vi "DT2.vi"(0 "input u(k)":dbl, 2 "Mode":enum16{"s-domain", "Frequency"}(ring), 5 "s-domain":cluster{"G":dbl, "T1":dbl, "T2":dbl}, 9 "frequency":cluster{"Td":dbl, "D":dbl, "f0":dbl}, 13 "initialize":bool) -> (8 "output y(k)":dbl)   [LabVIEW 2022 SP3]
uses:
  <vilib>/addons/Control Design/_Model Construction/Model Typedefs.llb/CD Transfer Function Model (SISO).ctl
  <vilib>/addons/Control Design/_Model Construction/NI_LinSys_Model Typedefs.lvlib
  <vilib>/addons/Control Design/_Model Construction/Model Typedefs.llb/CD General Elements.ctl
  <vilib>/addons/Control Design/_Model Construction/Model Typedefs.llb/CD Transfer Function Model (MIMO).ctl
  <vilib>/Simulation/DiscreteLinear/Implementation/NILVSim Discrete Transfer Function Direct.llb/SIM Discrete Transfer Function Diagram (SISO CD).vi
  <vilib>/Simulation/Implementation/XNodeFramework/SimXNode/SimX.xnode
  <vilib>/addons/Control Design/_Frequency Response Analysis/NI_CD_Frequency Response.lvlib
  <vilib>/addons/Control Design/_Frequency Response Analysis/Frequency Response.llb/Frequency Response subVI/cd_Bode (Transfer Function).vi
  <vilib>/addons/System Identification/Model Typedefs.llb/si_Bode Magnitude Plot.ctl
  <vilib>/addons/System Identification/NI_SysID.lvlib
  <vilib>/addons/System Identification/Model Typedefs.llb/si_Bode Phase Plot.ctl
panel:
  out "Bode Phase Plot":T1
  out "Bode Magnitude Plot":T2
  out "Step Response Graph":cluster{"time":dbl[], dbl[]}[](graph)
  out "S Transf":picture
  out "error out":errorcluster
  in  "error in (no error)":errorcluster
  out "element":T3 {"delay" format="%.4f"; "Denominator" format="%#_3g"; "Numerator" format="%#_3g"}
  out "Z Transf":picture
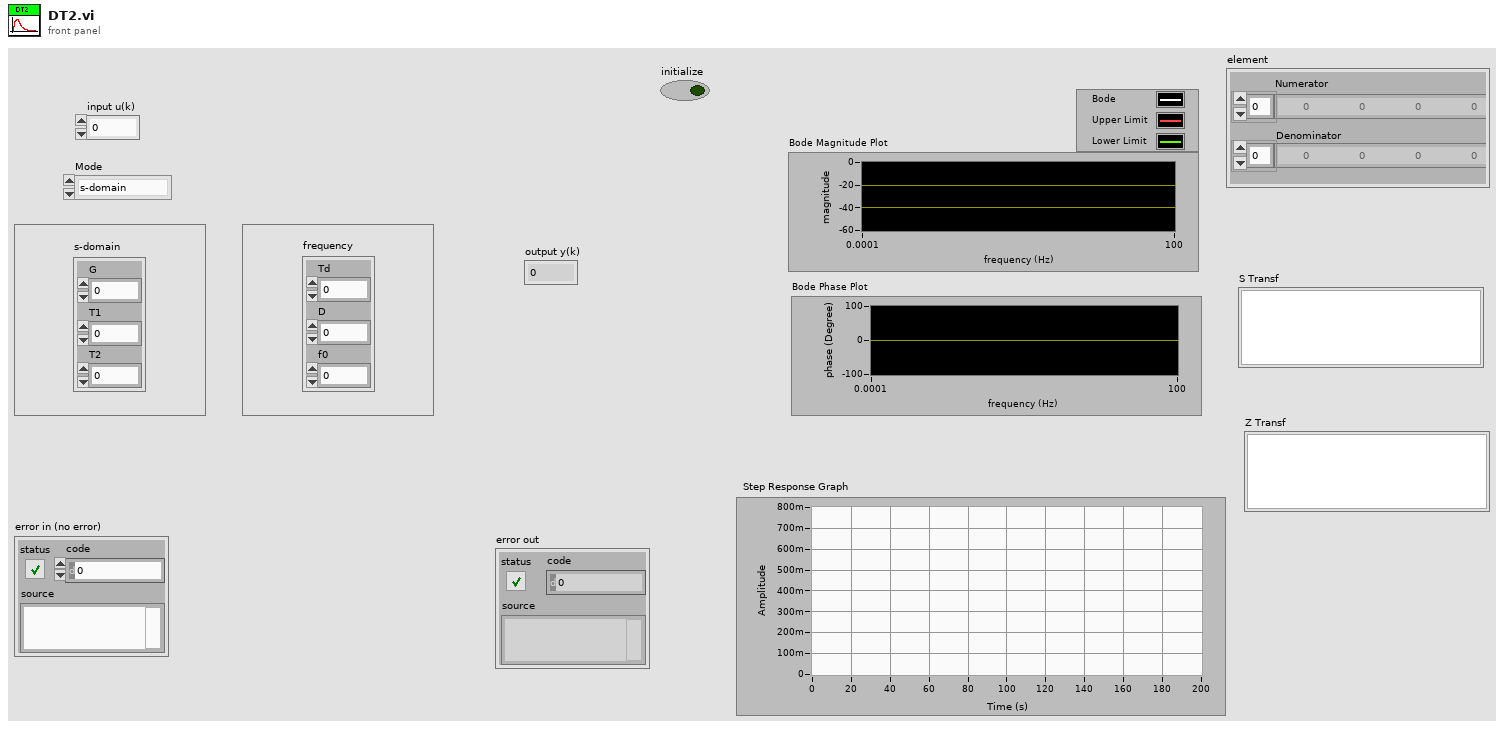
[diagram p1: front panel]
types:
  T1 = typedef "NI_SysID.lvlib/si_Bode Phase Plot.ctl" = cluster{"frequency":dbl[], "amplitude":dbl[]}[]
  T2 = typedef "NI_SysID.lvlib/si_Bode Magnitude Plot.ctl" = cluster{"frequency":dbl[], "amplitude":dbl[]}[]
  T3 = typedef "NI_LinSys_Model Typedefs.lvlib/CD Transfer Function Model (SISO).ctl" = cluster{"Numerator":dbl[], "Denominator":dbl[], "delay":dbl}
  T4 = typedef "NI_LinSys_Model Typedefs.lvlib/CD Transfer Function Model (MIMO).ctl" = cluster{"properties":T5, "transfer function(s)":T3[][]}
  T5 = typedef "NI_LinSys_Model Typedefs.lvlib/CD General Elements.ctl" = cluster{"Model name":string, "Input names":string[], "Output names":string[], "Input Delays":dbl[], "Output Delays":dbl[], "Sampling Time":dbl, "Notes":string}
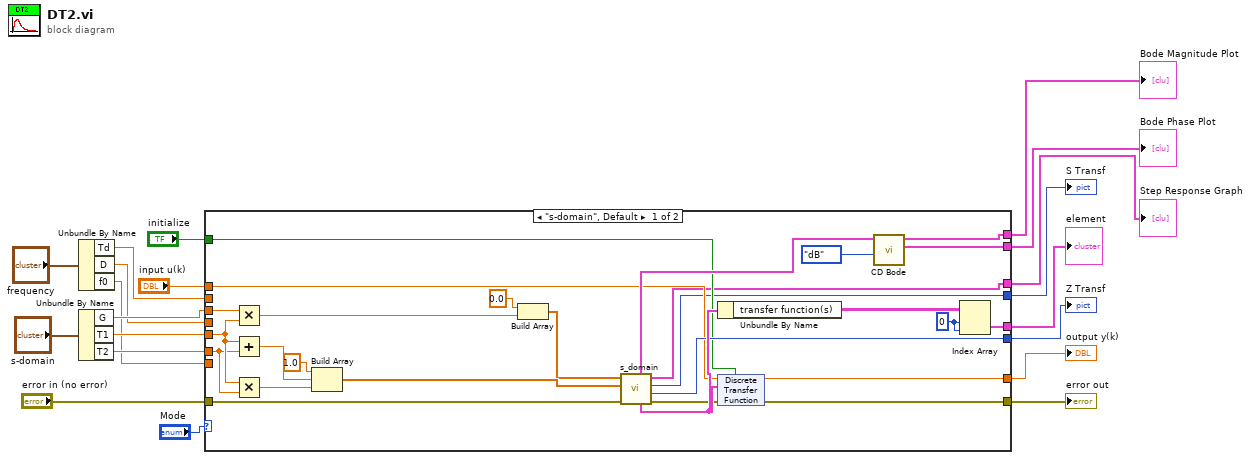
[diagram p0: block diagram]
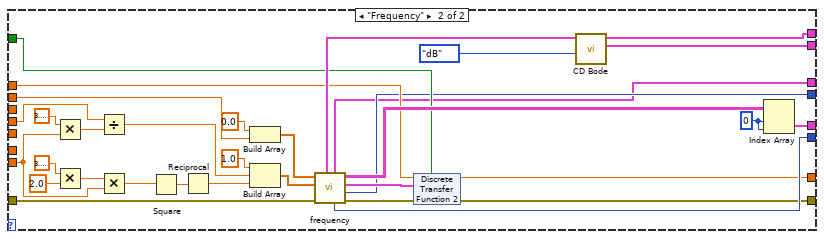
[diagram p2: hidden frame]
diagram:
  n1 = Unbundle By Name("frequency") -> ("Td"=w5:dbl, "D"=w4:dbl, "f0"=w3:dbl)
  n2 = Unbundle By Name("s-domain") -> ("G"=w9:dbl, "T1"=w8:dbl, "T2"=w7:dbl)
  n3 = case shown="\"s-domain\", Default" "Mode" {
    tunnel: [w34 w76] -> w19
    tunnel: [w33 w75] -> w18
    tunnel: "input u(k)" -> [w32 w73]
    tunnel: [w31 w74] -> w16
    tunnel: "error in (no error)" -> [w30 w72]
    tunnel: [w29 w71] -> w14
    tunnel: "initialize" -> [w28 w61]
    tunnel: [w27 w60] -> w12
    tunnel: [w26 w59] -> w11
    tunnel: w9 -> [w25 _]
    tunnel: w8 -> [w24 _]
    tunnel: w7 -> [w23 _]
    tunnel: w5 -> [_ w58]
    tunnel: w4 -> [_ w57]
    tunnel: w3 -> [_ w56]
    tunnel: [w22 w55] -> w2
    tunnel: [w21 w54] -> w1
    frame "s-domain", Default {
      w44 = 0 ("index (row)")
      n4 = Multiply(x=w25, y=w24) -> (x*y=w35:dbl)
      n5 = Add(x=w24, y=w23) -> (x+y=w39:dbl)
      n6 = Multiply(x=w24, y=w23) -> (x*y=w38:dbl)
      n7 = Build Array(1.0 ("element"), w39, w38) -> (w47:dbl[])
      n8 = Build Array(0.0 ("element"), w35) -> (w46:dbl[])
      n9 = call "s_domain.vi"("error in (no error)"=w30, "Denominator"=w47, "Numerator"=w46) -> ("error out"=w41:errorcluster, "z-domain"=w33:picture, "s-domain"=w27:picture, "Step Response Graph"=w26:cluster{"time":dbl[], dbl[]}[], "Discrete Transfer Function Model"=w42:T4, "Transfer Function Model"=w37:T4)  [unwired: 3 in]
      n10 = Unbundle By Name(w42) -> ("transfer function(s)"=w45:T3[][])
      n11 = xnode "Discrete Transfer Function"("input u(k)"=w32, "Transfer Function"=w42, "initialize"=w28, "error in (no error)"=w41) -> ("output y(k)"=w31:dbl, "error out"=w29:errorcluster)
      n12 = call-poly <vilib>:"CD Bode.vi"("Magnitude Scale"=enum16{"linear", "dB"}."dB", "Transfer Function Model"=w37) -> ("Bode Phase"=w21:cluster{"W":dbl[], "Magnitude":dbl[]}[], "Bode Magnitude"=w22:cluster{"W":dbl[], "Magnitude":dbl[]}[])  [unwired: 5 in, 3 out]
      n13 = Index Array(array=w45, index (row)=w44, index (col)=w44) -> (element=w34:T3)
    }
    frame "Frequency" {
      w83 = 0 ("index (row)")
      n14 = Multiply(x=3.141592653589793, y=w56) -> (x*y=w69:dbl)
      n15 = Multiply(x=3.141592653589793, y=2.0) -> (x*y=w65:dbl)
      n16 = Divide(x=w57, y=w69) -> (x/y=w68:dbl)
      n17 = Multiply(x=w65, y=w56) -> (x*y=w64:dbl)
      n18 = Square(x=w64) -> (x^2=w62:dbl)
      n19 = Reciprocal(x=w62) -> (1/x=w63:dbl)
      n20 = Build Array(0.0 ("element"), w58) -> (w85:dbl[])
      n21 = Build Array(1.0 ("element"), w68, w63) -> (w86:dbl[])
      n22 = call "frequency.vi"("error in (no error)"=w72, "Denominator"=w86, "Numerator"=w85) -> ("error out"=w80:errorcluster, "s-domain"=w60:picture, "Discrete Transfer Function Model"=w81:T4, "transfer function(s)"=w84:T3[][], "z-domain"=w75:picture, "Step Response Graph"=w59:cluster{"time":dbl[], dbl[]}[], "Transfer Function Model"=w78:T4)  [unwired: 2 in]
      n23 = xnode "Discrete Transfer Function 2"("input u(k)"=w73, "Transfer Function"=w81, "initialize"=w61, "error in (no error)"=w80) -> ("output y(k)"=w74:dbl, "error out"=w71:errorcluster)
      n24 = call-poly <vilib>:"CD Bode.vi"("Magnitude Scale"=enum16{"linear", "dB"}."dB", "Transfer Function Model"=w78) -> ("Bode Phase"=w54:cluster{"W":dbl[], "Magnitude":dbl[]}[], "Bode Magnitude"=w55:cluster{"W":dbl[], "Magnitude":dbl[]}[])  [unwired: 5 in, 3 out]
      n25 = Index Array(array=w84, index (row)=w83, index (col)=w83) -> (element=w76:T3)
    }
  }
  "element" <- w19
  "Z Transf" <- w18
  "output y(k)" <- w16
  "error out" <- w14
  "S Transf" <- w12
  "Step Response Graph" <- w11
  "Bode Magnitude Plot" <- w2
  "Bode Phase Plot" <- w1
